vi "Configure Digital Gen FFT Chirp.vi"(0 "VISA resource name":refnum<visa-resource-name>, 1 "Enable EQ Output Modification (T: Enable)":bool=TRUE, 2 "Enable Waveform (T: Enable)":bool=TRUE, 5 "Channel (0: chA)":i32(ring) items=["chA", "chB"], 7 "Amplitude (0 FFS)":dbl, 9 "FFT Source (0: csA0FFT)":i32(ring) items=["csA0FFT", "csA0FFT2Ch", "csA1FFT", "csA1FFT2Ch"], 11 "error in (no error)":errorcluster, 12 "Enable Variable Sweep (T: Enable)":bool=TRUE) -> (4 "VISA resource name out":refnum<visa-resource-name>, 15 "error out":errorcluster)   [LabVIEW 2014, in "Stanford Research SR1.lvlib"]
doc: "Configures the attributes for the Digital Generator FFT Chirp."
uses:
  Stanford Research SR1.lvlib
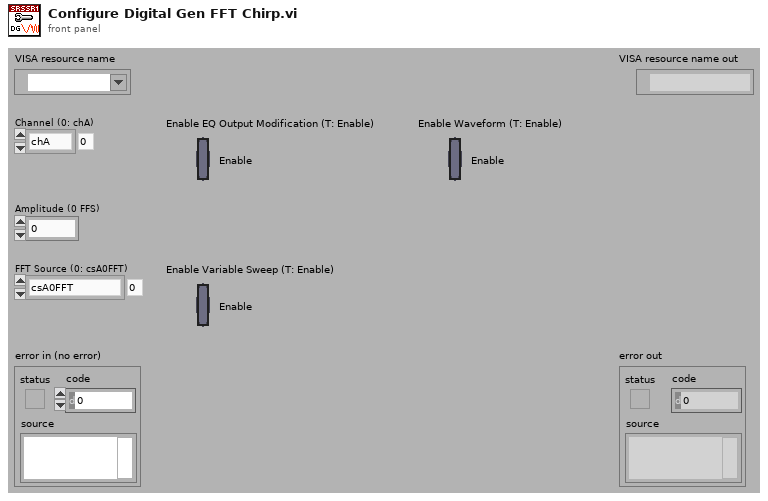
[diagram p1: front panel]
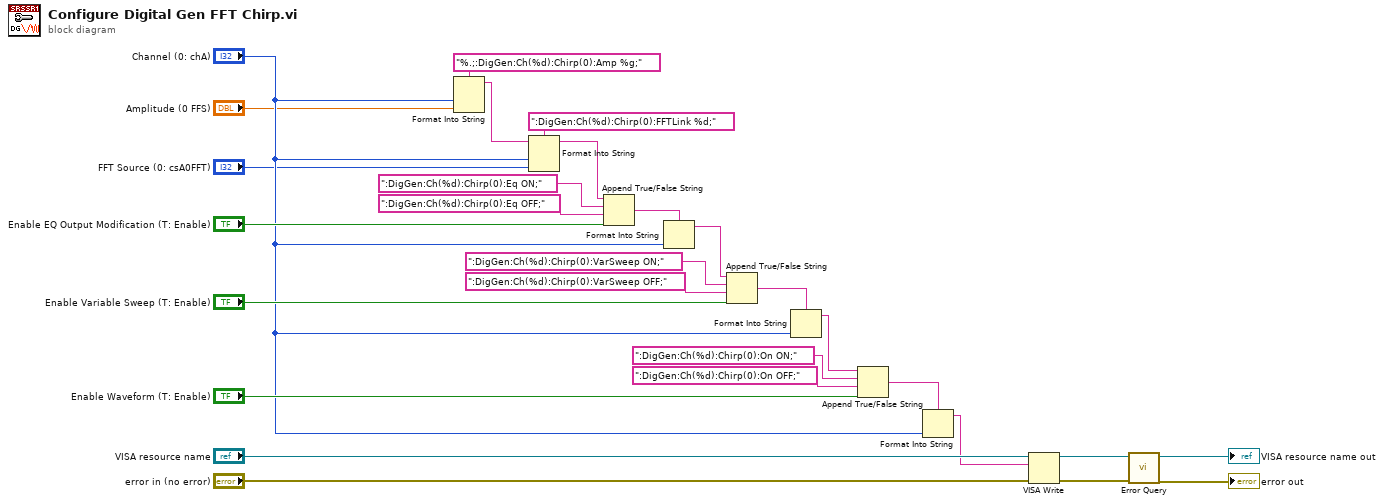
[diagram p0: block diagram]
diagram:
  n1 = Format Into String(format string="%.;:DigGen:Ch(%d):Chirp(0):Amp %g;", "Channel (0: chA)", "Amplitude (0 FFS)") -> (resulting string=w27:string)  [unwired: 2 in, 1 out]
  n2 = Format Into String(format string=":DigGen:Ch(%d):Chirp(0):FFTLink %d;", initial string=w27, "Channel (0: chA)", "FFT Source (0: csA0FFT)") -> (resulting string=w25:string)  [unwired: 1 in, 1 out]
  n3 = Append True/False String(1:"Enable EQ Output Modification (T: Enable)", 2:":DigGen:Ch(%d):Chirp(0):Eq OFF;", 3:":DigGen:Ch(%d):Chirp(0):Eq ON;", 4:w25) -> (0:w10:string)
  n4 = Format Into String(format string=w10, "Channel (0: chA)") -> (resulting string=w9:string)  [unwired: 2 in, 1 out]
  n5 = Append True/False String(1:"Enable Variable Sweep (T: Enable)", 2:":DigGen:Ch(%d):Chirp(0):VarSweep OFF;", 3:":DigGen:Ch(%d):Chirp(0):VarSweep ON;", 4:w9) -> (0:w7:string)
  n6 = Format Into String(format string=w7, "Channel (0: chA)") -> (resulting string=w6:string)  [unwired: 2 in, 1 out]
  n7 = Append True/False String(1:"Enable Waveform (T: Enable)", 2:":DigGen:Ch(%d):Chirp(0):On OFF;", 3:":DigGen:Ch(%d):Chirp(0):On ON;", 4:w6) -> (0:w5:string)
  n8 = Format Into String(format string=w5, "Channel (0: chA)") -> (resulting string=w4:string)  [unwired: 2 in, 1 out]
  n9 = VISA Write(VISA resource name="VISA resource name", write buffer=w4, error in (no error)="error in (no error)") -> (VISA resource name out=w14:refnum<visa-resource-name>, error out=w13:errorcluster)  [unwired: 1 out]
  n10 = call "Error Query.vi"("error in (no error)"=w13, "VISA resource name"=w14) -> ("error out"=→"error out":errorcluster, "VISA resource name out"=→"VISA resource name out":refnum<visa-resource-name>)  [unwired: 6 in, 2 out]
